vi "MFLI -- publish -- mfli handle.vi"(7 "publisher action":T2, 9 "Handle IN":T1 {"Handle" format="0x%08x"; "Conn" format="0x%08x"}) -> (1 "Handle Out":T1 {"Handle" format="0x%08x"; "Conn" format="0x%08x"})   [LabVIEW 2018]
uses:
  publisher action.ctl
  Applications/National Instruments/LabVIEW 2019 64-bit/instr.lib/Zurich Instruments LabOne/Public/ziTypeHandle.ctl
  Applications/National Instruments/LabVIEW 2019 64-bit/instr.lib/Zurich Instruments LabOne/Zurich Instruments LabOne.lvlib
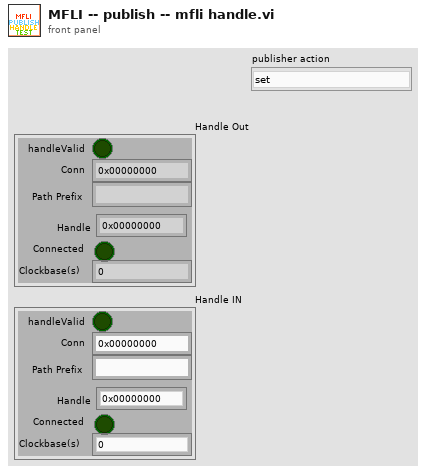
[diagram p1: front panel]
types:
  T1 = typedef "Zurich Instruments LabOne.lvlib/ziTypeHandle.ctl" = cluster{"handleValid":bool, "Conn":u64, "Path Prefix":string, "Handle":u64, "Connected":bool, "Clockbase(s)":dbl}
  T2 = typedef "publisher action.ctl" = enum16{"set", "get", "init", "check"}
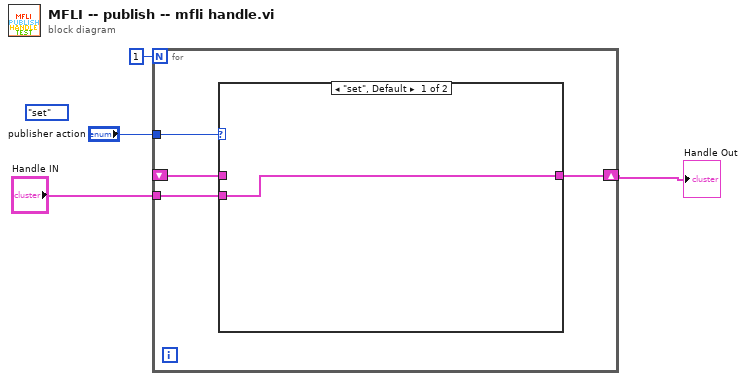
[diagram p0: block diagram]
diagram:
  (unwired) publisher_action."set" ("publisher action")
  n1 = for {
    N: 1 -> [_]
    tunnel: "publisher action" -> [w8]
    tunnel: "Handle IN" -> [w6]
    shift-right: [w7] -> w2
    shift-left: _ -> [w5]
    n2 = case shown="\"set\", Default" w8 {
      tunnel: [w9 w10] -> w7
      tunnel: w6 -> [w9 _]
      tunnel: w5 -> [_ w10]
      frame "set", Default {
      }
      frame "get" {
      }
    }
  }
  "Handle Out" <- w2
